vi "PCO_SetTimestampMode.vi"(8 "error in (no error)":errorcluster {"code" format="%x"}, 10 "wTimeStampMode":u16(ring) items=["OFF", "Binary", "Binary+ASCII", "ASCII"], 11 "ph":u64) -> (0 "error out":errorcluster {"code" format="%x"}, 2 "ErrorMessage":i32 format="%x", 3 "ph out":u64)   [LabVIEW 2019, in "SDK.lvlib" / "RecordingControl.lvlib"]
doc: "<b>Description:</b>\nThis function does set the timestamp mode of the camera. Details about the timestamp modes are explained in the previous command PCO_GetTimestampMode.\n\n<b>Supported camera type:</b>\nAll cameras\n\n<b>Descriptor dependency:</b>\ndwGeneralCapsDESC1: NO_TIMESTAMP"
uses:
  RecordingControl.lvlib
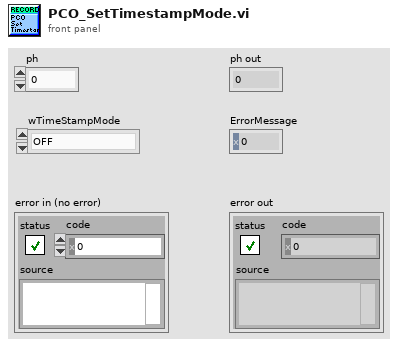
[diagram p1: front panel]
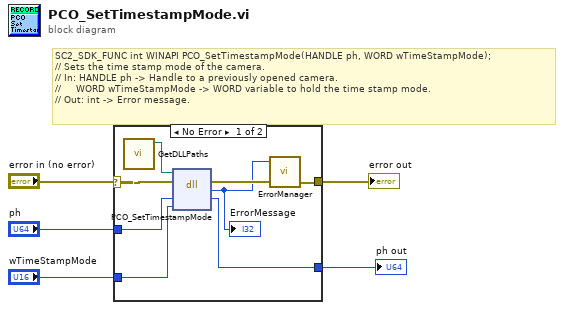
[diagram p0: block diagram]
diagram:
  # "SC2_SDK_FUNC int WINAPI PCO_SetTimestampMode(HANDLE ph, WORD wTimeStampMode);\n// Sets the time stamp mode of the camera.\n// In: HANDLE ph -> Handle to a previously opened camera.\n//     WORD wTimeStampMode -> WORD variable to hold the time stamp mode.\n// Out: int -> Error message."
  n1 = case shown="No Error" "error in (no error)" {
    selector: "error in (no error)" -> [w10 w15]
    tunnel: "ph" -> [w13 w14]
    tunnel: [w12 w14] -> w4
    tunnel: "wTimeStampMode" -> [w11 _]
    tunnel: [w8 w15] -> w2
    frame No Error {
      n2 = call "GetDLLPaths.vi"() -> ("SC2_Cam_Path"=w6:path)  [unwired: 9 in, 2 out]
      n3 = dll-call lib="?" fn="PCO_SetTimestampMode"(path in=w6, error in=w10, "ph"=w13, "wTimeStampMode"=w11) -> (error out=w9:errorcluster, "return type"=w7:i32, "ph"=w12:u64)  [unwired: 2 in, 1 out]
      "ErrorMessage" <- w7
      n4 = call "ErrorManager.vi"("error in (no error)"=w9, "error code"=w7) -> ("error out"=w8:errorcluster)  [unwired: 3 in]
    }
    frame Error {
    }
  }
  "ph out" <- w4
  "error out" <- w2
